vi "Configure Modulation(QPSK).vi"(0 "VISA resource name":refnum<visa-resource-name>, 1 "Enable QPSK Modulation (F: Disable)":bool, 2 "Phase 3 (225 Degree)":dbl=225.0, 5 "Channel (1: Channel 1)":i32(ring)=1 items=["Channel 1"=1, "Channel 2"=2], 7 "QPSK Source (0: PN15)":i32(ring) items=["PN15", "PN21"], 9 "Phase 1 (45 Degree)":dbl=45.0, 11 "error in (no error)":errorcluster, 12 "Phase 2 (135 Degree)":dbl=135.0, 13 "QPSK Rate (100 Hz)":dbl=100.0) -> (4 "VISA resource name out":refnum<visa-resource-name>, 15 "error out":errorcluster)   [LabVIEW 2012, in "RIGOL DG4000 Series.lvlib"]
doc: "Configures QPSK (Quadrature Phase Shift Keying) modulation."
uses:
  <instrlib>/RIGOL DG4000 Series/RIGOL DG4000 Series.lvlib
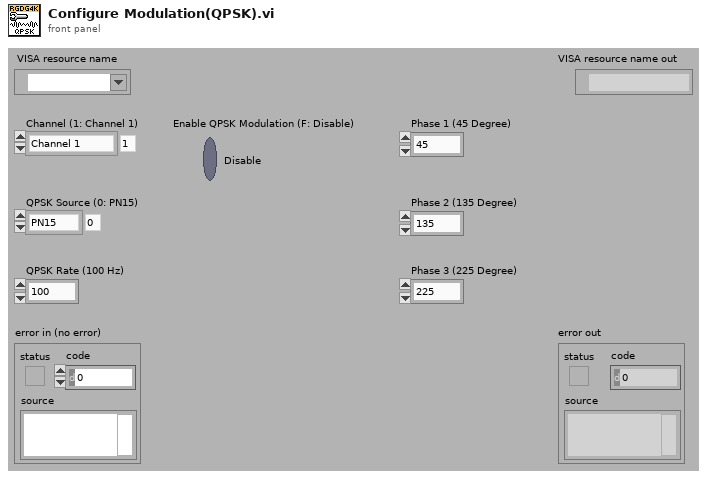
[diagram p1: front panel]
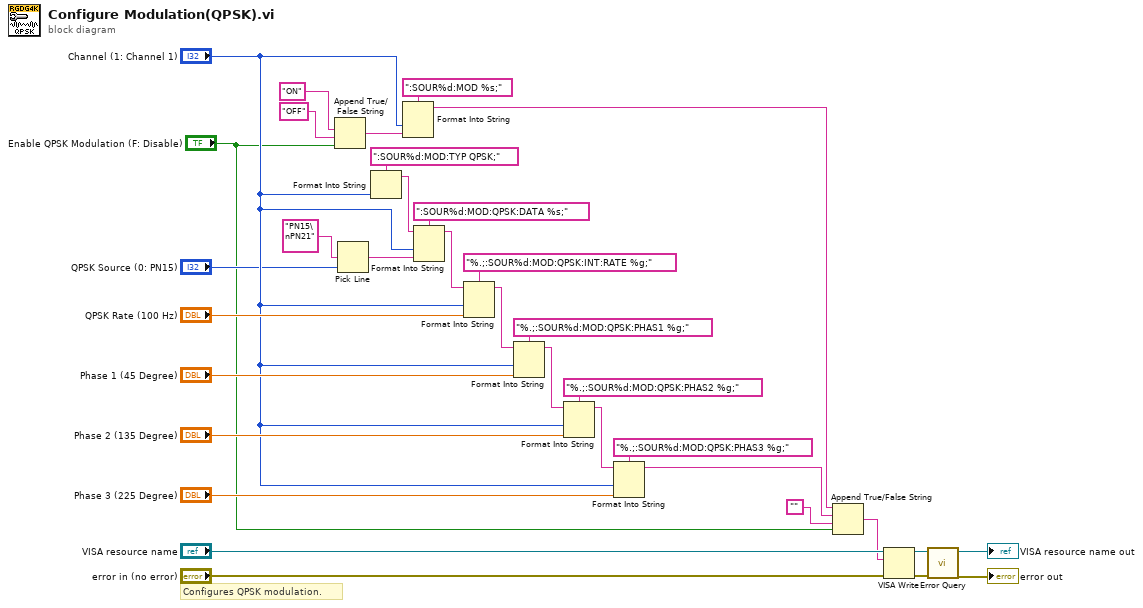
[diagram p0: block diagram]
diagram:
  # "Configures QPSK modulation."
  n1 = Append True/False String(1:"Enable QPSK Modulation (F: Disable)", 2:"OFF", 3:"ON") -> (0:w31:string)  [unwired: 1 out]
  n2 = Pick Line(multi-line string="PN15\nPN21", line index="QPSK Source (0: PN15)") -> (output string=w7:string)  [unwired: 1 out]
  n3 = Format Into String(format string=":SOUR%d:MOD:TYP QPSK;", "Channel (1: Channel 1)") -> (resulting string=w29:string)  [unwired: 2 in, 1 out]
  n4 = Format Into String(format string=":SOUR%d:MOD %s;", "Channel (1: Channel 1)", w31) -> (resulting string=w4:string)  [unwired: 2 in, 1 out]
  n5 = Format Into String(format string=":SOUR%d:MOD:QPSK:DATA %s;", initial string=w29, "Channel (1: Channel 1)", w7) -> (resulting string=w27:string)  [unwired: 1 in, 1 out]
  n6 = Format Into String(format string="%.;:SOUR%d:MOD:QPSK:INT:RATE %g;", initial string=w27, "Channel (1: Channel 1)", "QPSK Rate (100 Hz)") -> (resulting string=w24:string)  [unwired: 1 in, 1 out]
  n7 = Format Into String(format string="%.;:SOUR%d:MOD:QPSK:PHAS1 %g;", initial string=w24, "Channel (1: Channel 1)", "Phase 1 (45 Degree)") -> (resulting string=w21:string)  [unwired: 1 in, 1 out]
  n8 = Format Into String(format string="%.;:SOUR%d:MOD:QPSK:PHAS2 %g;", initial string=w21, "Channel (1: Channel 1)", "Phase 2 (135 Degree)") -> (resulting string=w18:string)  [unwired: 1 in, 1 out]
  n9 = Format Into String(format string="%.;:SOUR%d:MOD:QPSK:PHAS3 %g;", initial string=w18, "Channel (1: Channel 1)", "Phase 3 (225 Degree)") -> (resulting string=w3:string)  [unwired: 1 in, 1 out]
  n10 = Append True/False String(1:"Enable QPSK Modulation (F: Disable)", 2:"", 3:w3, 4:w4) -> (0:w1:string)
  n11 = VISA Write(VISA resource name="VISA resource name", write buffer=w1, error in (no error)="error in (no error)") -> (VISA resource name out=w13:refnum<visa-resource-name>, error out=w12:errorcluster)  [unwired: 1 out]
  n12 = call <instrlib>:"Error Query.vi"("error in (no error)"=w12, "VISA resource name"=w13) -> ("error out"=→"error out":errorcluster, "VISA resource name out"=→"VISA resource name out":refnum<visa-resource-name>)  [unwired: 8 out]
